vi "Share Trigger.vi"(4 "trigger delay":dbl caption="trigger delay (0)" format="%.4f", 6 "trigger holdoff":dbl caption="trigger holdoff (0)" format="%.4f", 7 "trigger slope":T2 caption="trigger slope (Positive)", 8 "error in":errorcluster, 10 "shared terminal":T1="VAL_RTSI_0" caption="output terminal (PXI Trig 0)", 11 "instrument handles":refnum<k15>[](array[refnum])) -> (0 "error out":errorcluster, 3 "instrument handles out":refnum<k15>[](array[refnum]))   [LabVIEW 2020, in "varilib.lvlib"]
doc: "Export trigger from first device into all other devices in \"instrument handles\" array. Thus only first device has to be triggered to start sampling on all devices."
uses:
  varilib.lvlib
  <instrlib>/niScope/Controls/niScope exportable signals.ctl
  <instrlib>/niScope/Configure/Trigger/niScope Configure Trigger Digital.vi
  <instrlib>/niScope/Controls/niScope export destinations.ctl
  <instrlib>/niScope/Controls/niScope trigger slope.ctl
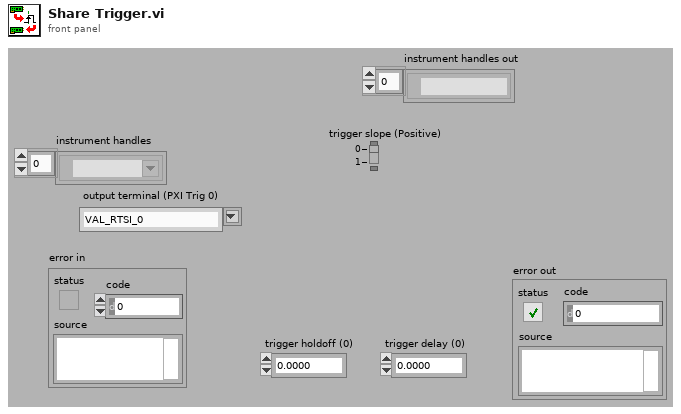
[diagram p1: front panel]
types:
  T1 = typedef "niScope export destinations.ctl" = string
  T2 = typedef "niScope trigger slope.ctl" = i32
  T3 = typedef "niScope exportable signals.ctl" = u16
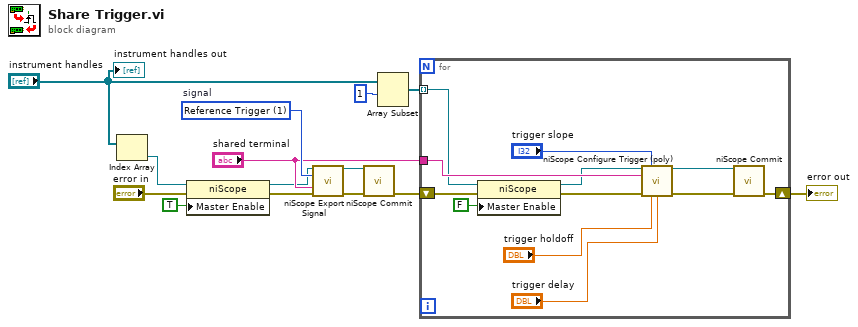
[diagram p0: block diagram]
diagram:
  w14 = T3 1 items=["Start Trigger"=2, "Advance Trigger"=5, "Reference Trigger"=1, "End of Record Event"=4, "End of Acquisition Event"=3, "Ready for Start Event"=7, "Ready for Advance Event"=6, "Ready for Reference Event"=10, "Reference Clock"=100, "Sample Clock"=101]  # signal
  n1 = Index Array(array="instrument handles") -> (element=w6:refnum<k15>)  [unwired: 1 in]
  n2 = property class="niScope"(reference=w6, error in="error in", "Master Enable"=TRUE ("Synchronization:Master Enable")) -> (reference out=w5:refnum<k15>, error out=w2:errorcluster)
  n3 = call <instrlib>:"niScope Export Signal.vi"("instrument handle"=w5, "signal"=w14, "output terminal"="shared terminal", "error in"=w2) -> ("instrument handle out"=w4:refnum<k15>, "error out"=w1:errorcluster)  [unwired: 10 in]
  n4 = call <instrlib>:"niScope Commit.vi"("instrument handle"=w4, "error in"=w1) -> ("error out"=w12:errorcluster)  [unwired: 12 in, 1 out]
  n5 = Array Subset(array="instrument handles", index=1) -> (w9:refnum<k15>[])  [unwired: 1 in]
  n6 = for {
    tunnel: w9 -> [w15] mode=indexing
    tunnel: "shared terminal" -> [w24]
    shift-right: [w23] -> w7
    shift-left: w12 -> [w20]
    n7 = property class="niScope"(reference=w15, error in=w20, "Master Enable"=FALSE ("Synchronization:Master Enable")) -> (reference out=w17:refnum<k15>, error out=w19:errorcluster)
    n8 = call-poly <instrlib>:"niScope Configure Trigger (poly).vi"("instrument handle"=w17, "trigger slope"="trigger slope", "trigger source"=w24, "error in"=w19, "trigger holdoff"="trigger holdoff", "trigger delay"="trigger delay") -> ("instrument handle out"=w16:refnum<k15>, "error out"=w18:errorcluster)  [unwired: 8 in]
    n9 = call <instrlib>:"niScope Commit.vi"("instrument handle"=w16, "error in"=w18) -> ("error out"=w23:errorcluster)  [unwired: 12 in, 1 out]
  }
  "error out" <- w7
  "instrument handles out" <- "instrument handles"
